vi "SUB_Decrypt.vi"(0 "encrypt Filename":string) -> (1 "Decrypted Output":string, 3 "Ok ?":bool)   [LabVIEW 2011]
doc: "This VI usea the System.Security.Cryptography.DESCryptoServiceProvider class, provided by the .NET 1.1 framework in the mscorlib.dll, for data encryption and decryption. This VI uses the Initialization Vector (IV) and the secret key used for the Data Encryption Standard (DES) algorithm to decrypt the data. The correct IV and key are necessary to decrypt the information\n\nYou can obtain the values of the constants used for the methods using the Microsoft Intermediate language Disassembler (ILDasm.exe). This tool installs with the Microsoft .NET 1.1 framework SDK.\n\nRefer to the Microsoft Developers Network at http://msdn.microsoft.com for more information about the mehods and properties of the methods and properties used in this VI."
panel:
  out "File Existing True/Flase":bool
  out "code":i32
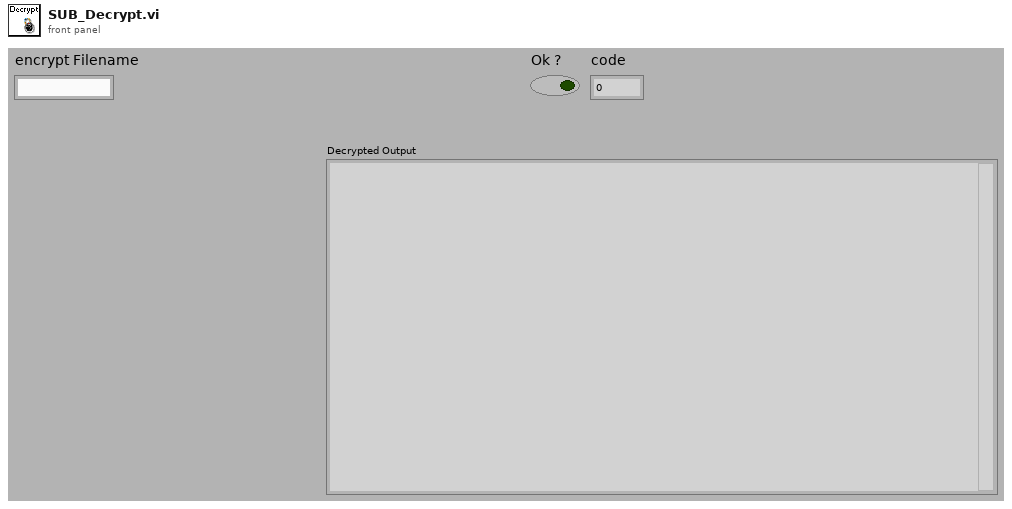
[diagram p1: front panel]
types:
  T1 = enum32{"invalid app kind", "Development System", "Run Time System", "Student Edition", "Embedded LabVIEW", "Evaluation", "Custom"}
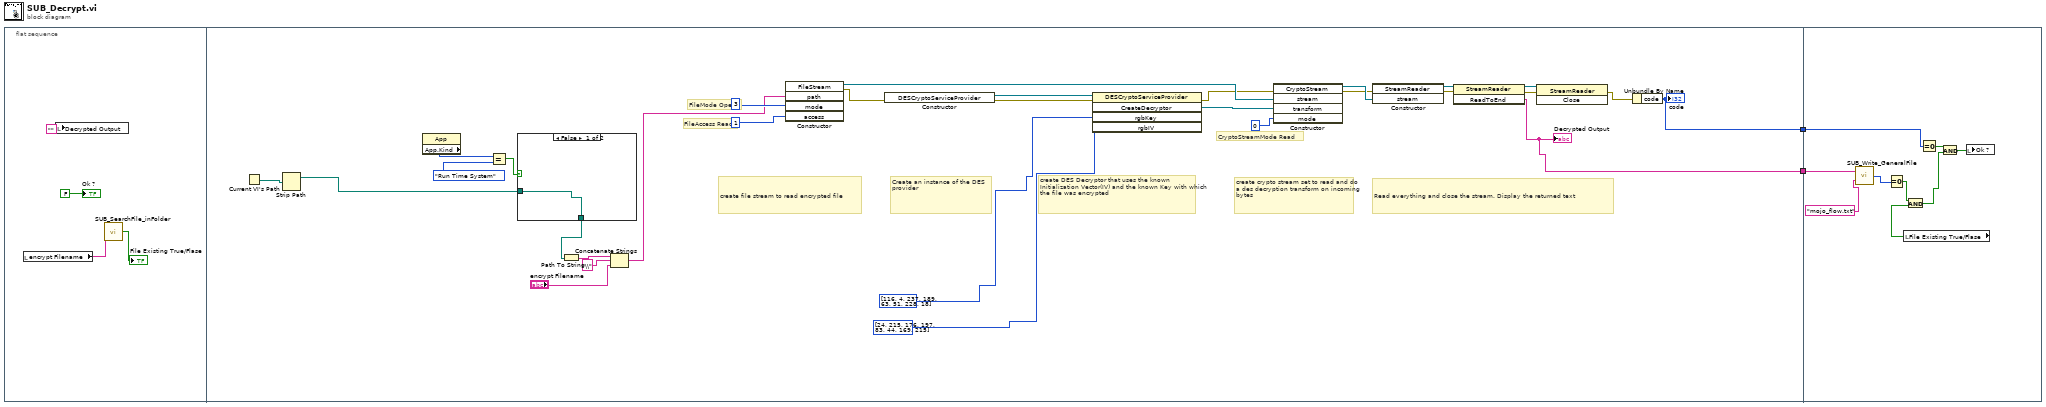
[diagram p0: block diagram]
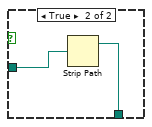
[diagram p2: hidden frame]
diagram:
  n1 = flat-sequence {
    tunnel: [w10] -> w2
    tunnel: [w9] -> w1
    tunnel: w2 -> [w41]
    tunnel: w1 -> [w40]
    frame #0 {
      n2 = local read "encrypt Filename"() -> (w4:string)
      n3 = local write "Decrypted Output"("") -> ()
      n4 = call "SUB_SearchFile_inFolder.vi"("Search Filename in Folder"=w4) -> ("File Existing True/Flase"=→"File Existing True/Flase":bool)  [unwired: 1 in]
      "Ok ?" <- FALSE
    }
    frame #1 {
      # "Read everything and close the stream. Display the returned text"
      # "create crypto stream set to read and do a des decryption transform on incoming bytes"
      # "create DES Decryptor that uses the known Initialization Vector(IV) and the known Key with which the file was encrypted"
      # "Create an instance of the DES provider"
      # "create file stream to read encrypted file"
      # "CryptoStreamMode Read"
      # "FileAccess Read"
      # "FileMode Open"
      n5 = Current VI's Path() -> (path=w21:path)
      n6 = Strip Path(path=w21) -> (stripped path=w17:path)  [unwired: 1 out]
      n7 = property class="App"() -> ("App.Kind"=w20:T1)  [unwired: 2 in, 2 out]
      n8 = Equal?(x=w20, y=T1."Run Time System" ("Application:Kind")) -> (x = y?=w18:bool)
      n9 = case shown="False" w18 {
        tunnel: w17 -> [w37 w39]
        tunnel: [w37 w38] -> w16
        frame False {
        }
        frame True {
          n10 = Strip Path(path=w39) -> (stripped path=w38:path)  [unwired: 1 out]
        }
      }
      n11 = Path To String(path=w16) -> (string=w15:string)
      n12 = Concatenate Strings(w15, "\\" ("string"), "encrypt Filename") -> (w12:string)
      n13 = constructor class="FileStream"("path"=w12, "mode"=3, "access"=1) -> (reference out=w32:refnum<k24>, error out=w22:errorcluster)  [unwired: 3 in, 4 out]
      n14 = constructor class="DESCryptoServiceProvider"(error in=w22) -> (reference out=w36:refnum<k24>, error out=w35:errorcluster)  [unwired: 2 in, 1 out]
      n15 = invoke class="DESCryptoServiceProvider" method="CreateDecryptor"(reference=w36, error in=w35, "rgbKey"=u8[] [116, 4, 237, 189, 63, 51, 228, 18] ("Key"), "rgbIV"=u8[] [24, 215, 176, 197, 83, 44, 169, 215] ("IV")) -> (error out=w23:errorcluster, "CreateDecryptor"=w31:refnum<k24>)  [unwired: 1 in, 3 out]
      n16 = constructor class="CryptoStream"(error in=w23, "stream"=w32, "transform"=w31, "mode"=0) -> (reference out=w29:refnum<k24>, error out=w26:errorcluster)  [unwired: 2 in, 4 out]
      n17 = constructor class="StreamReader"(error in=w26, "stream"=w29) -> (reference out=w28:refnum<k24>, error out=w27:errorcluster)  [unwired: 2 in, 2 out]
      n18 = invoke class="StreamReader" method="ReadToEnd"(reference=w28, error in=w27) -> (reference out=w25:refnum<k24>, error out=w24:errorcluster, "ReadToEnd"=w10:string)  [unwired: 1 in]
      "Decrypted Output" <- w10
      n19 = invoke class="StreamReader" method="Close"(reference=w25, error in=w24) -> (error out=w11:errorcluster)  [unwired: 1 in, 2 out]
      n20 = Unbundle By Name(w11) -> ("code"=w9:i32)
      "code" <- w9
    }
    frame #2 {
      n21 = call "SUB_Write_GeneralFile.vi"("Filename"="mojo_flow.txt", "Text Input"=w41) -> ("err code"=w45:i32)
      n22 = Equal To 0?(x=w45) -> (x = 0?=w46:bool)
      n23 = local read "File Existing True/Flase"() -> (w47:bool)
      n24 = And(x=w46, y=w47) -> (x .and. y?=w48:bool)
      n25 = Equal To 0?(x=w40) -> (x = 0?=w43:bool)
      n26 = And(x=w43, y=w48) -> (x .and. y?=w44:bool)
      n27 = local write "Ok ?"(w44) -> ()
    }
  }
